vi "Translate Position to Grid.vi"(11 "Obstacle Avoidance Data":T1) -> (3 "Obstactle Avoidance Data":T1)   [LabVIEW 2017]
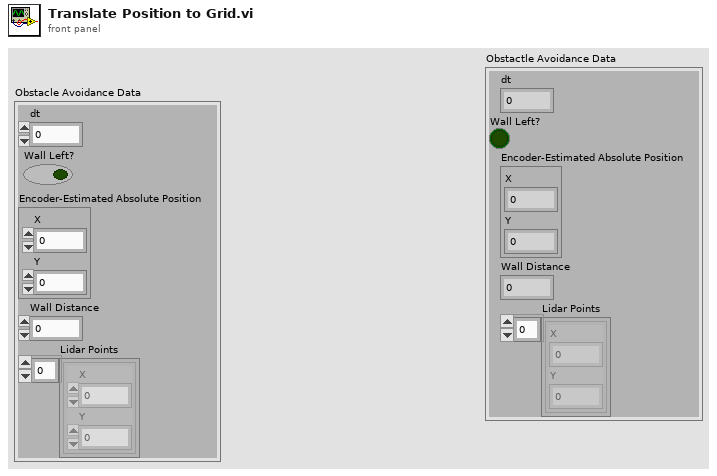
[diagram p1: front panel]
types:
  T1 = cluster{"dt":dbl, "Wall Left?":bool, "Encoder-Estimated Absolute Position":cluster{"X":dbl, "Y":dbl}, "Wall Distance":dbl, "Lidar Points":cluster{"X":dbl, "Y":dbl}[]}
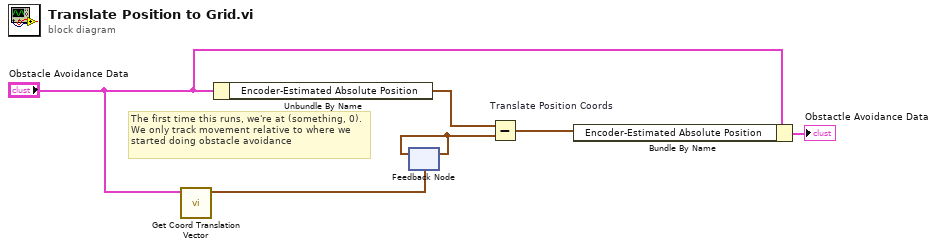
[diagram p0: block diagram]
diagram:
  # "The first time this runs, we're at (something, 0). We only track movement relative to where we started doing obstacle avoidance"
  n1 = call "Get Coord Translation Vector.vi"("Obstacle Avoidance Data"="Obstacle Avoidance Data") -> ("Translation Vector"=w5:cluster{"X":dbl, "Y":dbl})  [unwired: 10 in]
  n2 = Unbundle By Name("Obstacle Avoidance Data") -> ("Encoder-Estimated Absolute Position"=w4:cluster{"X":dbl, "Y":dbl})
  n3 = feedback #1(w5) -> (w6:cluster{"X":dbl, "Y":dbl})
  n4 = feedback-in #1(w6) -> ()
  n5 = Subtract "Translate Position Coords"(x=w4, y=w6) -> (x-y=w3:cluster{"X":dbl, "Y":dbl})
  n6 = Bundle By Name(cluster="Obstacle Avoidance Data", "Encoder-Estimated Absolute Position"=w3) -> (→"Obstactle Avoidance Data":T1)
